vi "File.Search Folder.vi"(9 "Search Pattern":string, 10 "Folders":path[](array[path]), 11 "Files In":path[](array[path])) -> (2 "SubFolders":path[](array[path]), 3 "Files Out":path[](array[path]))   [LabVIEW 2018]
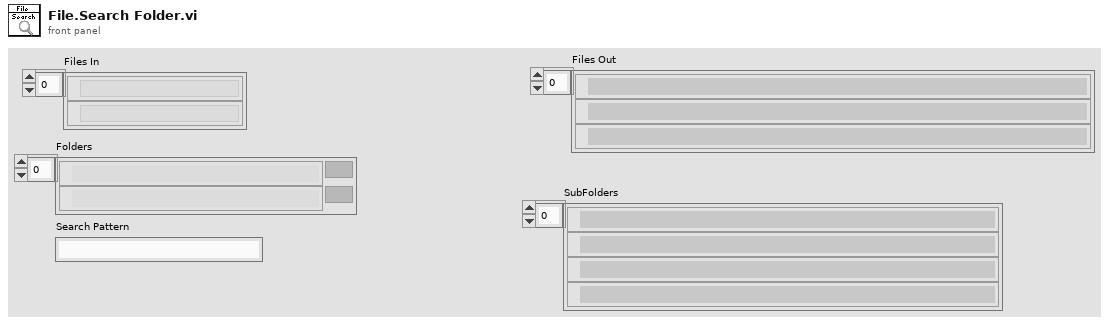
[diagram p1: front panel]
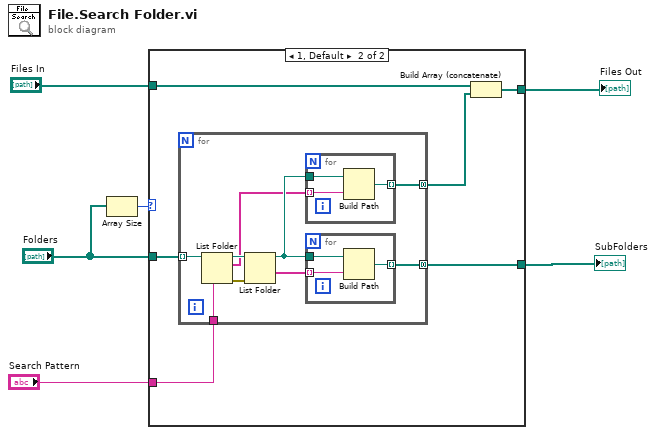
[diagram p0: block diagram]
diagram:
  n1 = Array Size(array="Folders") -> (size(s)=w3:i32)
  n2 = case shown="1, Default" w3 {
    tunnel: "Search Pattern" -> [_ w13]
    tunnel: [_ w12] -> w5
    tunnel: "Folders" -> [_ w11]
    tunnel: "Files In" -> [w7 w9]
    tunnel: [w7 w8] -> w1
    frame 0 {
    }
    frame 1, Default {
      n3 = for {
        tunnel: w11 -> [w17] mode=indexing
        tunnel: [w20] -> w12 mode=concatenating
        tunnel: [w19] -> w10 mode=concatenating
        tunnel: w13 -> [w15]
        n4 = List Folder(path=w17, pattern=w15) -> (path out=w16:path, filenames=w14:string[], error out=w18:errorcluster)  [unwired: 2 in, 1 out]
        n5 = List Folder(path=w16, error in=w18) -> (path out=w21:path, folder names=w22:string[])  [unwired: 2 in, 2 out]
        n6 = for {
          tunnel: w14 -> [w27] mode=indexing
          tunnel: w21 -> [w28]
          tunnel: [w26] -> w19 mode=indexing
          n7 = Build Path(base path=w28, name or relative path=w27) -> (appended path=w26:path)
        }
        n8 = for {
          tunnel: w22 -> [w24] mode=indexing
          tunnel: w21 -> [w25]
          tunnel: [w23] -> w20 mode=indexing
          n9 = Build Path(base path=w25, name or relative path=w24) -> (appended path=w23:path)
        }
      }
      n10 = Build Array (concatenate)(w9, w10) -> (w8:path[])
    }
  }
  "SubFolders" <- w5
  "Files Out" <- w1
